vi "get_period.vi"(8 "error in (no error)":errorcluster, 11 "GenericClock in":refnum<class "GenericClock.lvclass">) -> (0 "error out":errorcluster, 2 "period":dbl[unit], 3 "GenericClock out":refnum<class "GenericClock.lvclass">)   [LabVIEW 2010, in "GenericClock.lvclass"]
uses:
  GenericClock.lvclass
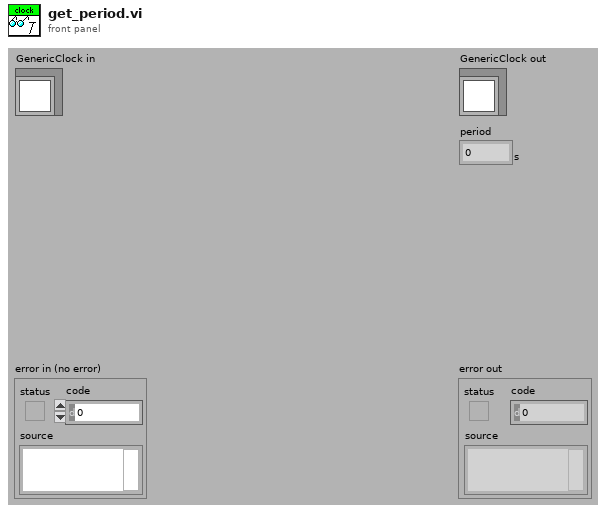
[diagram p1: front panel]
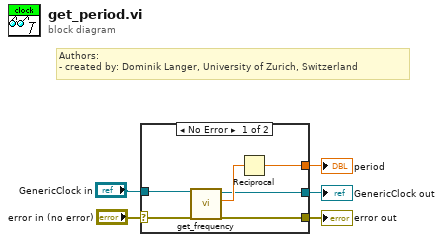
[diagram p0: block diagram]
diagram:
  # "Authors: \n- created by: Dominik Langer, University of Zurich, Switzerland"
  n1 = case shown="No Error" "error in (no error)" {
    selector: "error in (no error)" -> [w10 w13]
    tunnel: [w9 w13] -> w4
    tunnel: [w7 w12] -> w2
    tunnel: "GenericClock in" -> [w8 w12]
    tunnel: [w6 _] -> w1
    frame No Error {
      n2 = call-dynamic "get_frequency.vi"("error in (no error)"=w10, "GenericClock.lvclass in"=w8) -> ("error out"=w9:errorcluster, "frequency"=w11:dbl[unit], "GenericClock.lvclass out"=w7:refnum<class "GenericClock.lvclass">)  [unwired: 7 out]
      n3 = Reciprocal(x=w11) -> (1/x=w6:dbl[unit])
    }
    frame Error {
    }
  }
  "error out" <- w4
  "GenericClock out" <- w2
  "period" <- w1
